vi "Init from Ref.vi"(10 "Cell View .NET":refnum<k24>, 11 "Cell View in":refnum<class "Cell View.lvclass">) -> (3 "Cell View out":refnum<class "Cell View.lvclass">)   [LabVIEW 2023, in "SourceGrid.lvlib" / "Cell View.lvclass"]
uses:
  Cell View.lvclass
  D:/git/Sourcegrid-LabVIEW/dll/SourceGrid.dll
  dll/SourceGrid.dll
  Cell View.lvclass/Cell View.ctl
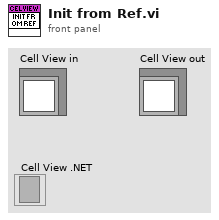
[diagram p1: front panel]
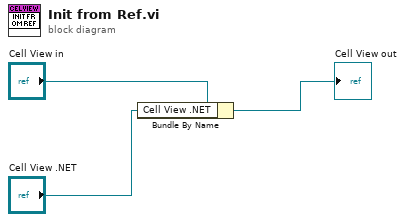
[diagram p0: block diagram]
diagram:
  n1 = Bundle By Name(cluster="Cell View in", "Cell View .NET"="Cell View .NET") -> (→"Cell View out":refnum<class "Cell View.lvclass">)
